vi "~ExampleCluster.vi"() -> ()   [LabVIEW 2017]
uses:
  Users/chris clark/Documents/Bolder/SEAKR/OBP/Product_Development/ULIP_SFP/LoopBackUtility/LoopbackToolClasses/ConfigMgr_N-ReceiverSubvis/Properties_N-Receiver.ctl
panel:
  in  "Replace? (F)":bool
  out "DefaultProperties out":T1={"Network"={"Local IP Address"="", "FPGA IP Address"="", "Local UDP Listener Port"=50000, "Destination UDP Port"=64880, "Rx Listener Timeout, ms"=0, "Receive Buffer Size"=8192, "Send Buffer Size"=512, "RemoteIPAddresses"=[]}, "TX Properties"={"Interpacket Gap, ms"=1, "Insert gap (N)"=1, "Packet.TxType"=0, "Packet.MaxLen"=8968, "Packet.MinLen"=7000}} {"TX Properties"."Packet.TxType" items=["Fixed", "Variable"]}
  in  "Write=True":bool
  in  "CfgFilePath":path=path "C:/dummy/testCluzzterz.ini"
  out "error out 2":errorcluster
  in  "DefaultProperties":T1={"Network"={"Local IP Address"="", "FPGA IP Address"="", "Local UDP Listener Port"=50000, "Destination UDP Port"=64880, "Rx Listener Timeout, ms"=0, "Receive Buffer Size"=8192, "Send Buffer Size"=512, "RemoteIPAddresses"=[]}, "TX Properties"={"Interpacket Gap, ms"=1, "Insert gap (N)"=1, "Packet.TxType"=0, "Packet.MaxLen"=8968, "Packet.MinLen"=7000}} {"TX Properties"."Packet.TxType" items=["Fixed", "Variable"]}
  # "Replace=True blows away\nold array values (deletes\nsections before writing)"
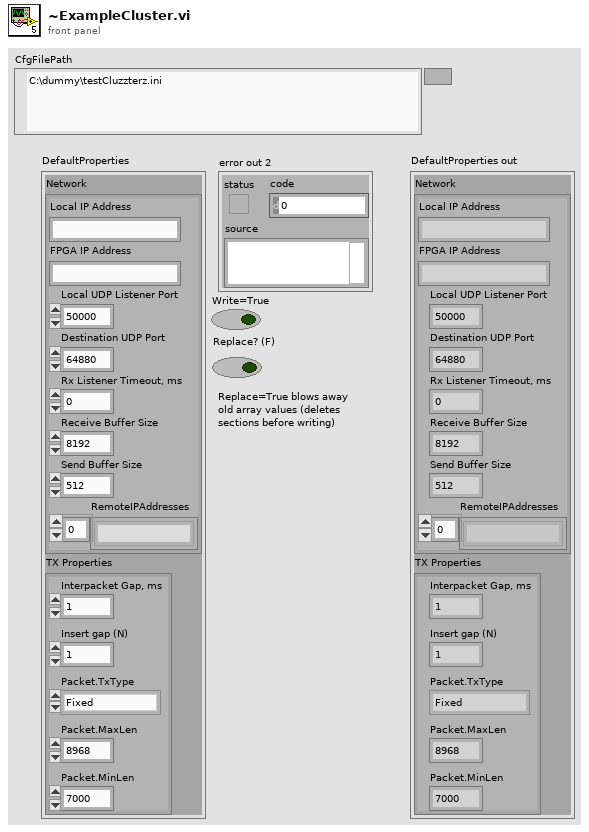
[diagram p1: front panel]
types:
  T1 = typedef "Properties_N-Receiver.ctl" = cluster{"Network":cluster{"Local IP Address":string, "FPGA IP Address":string, "Local UDP Listener Port":u16, "Destination UDP Port":u16, "Rx Listener Timeout, ms":i32, "Receive Buffer Size":u32, "Send Buffer Size":u32, "RemoteIPAddresses":string[]}, "TX Properties":cluster{"Interpacket Gap, ms":u32, "Insert gap (N)":i32, "Packet.TxType":i32, "Packet.MaxLen":i32, "Packet.MinLen":i32}}
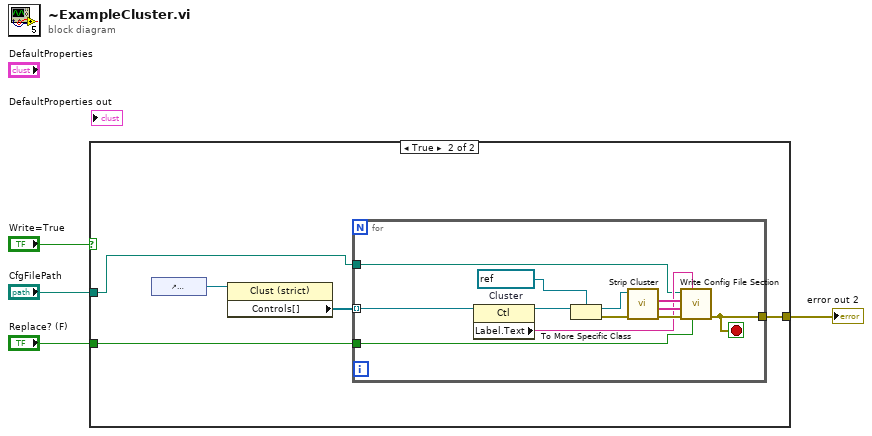
[diagram p0: block diagram]
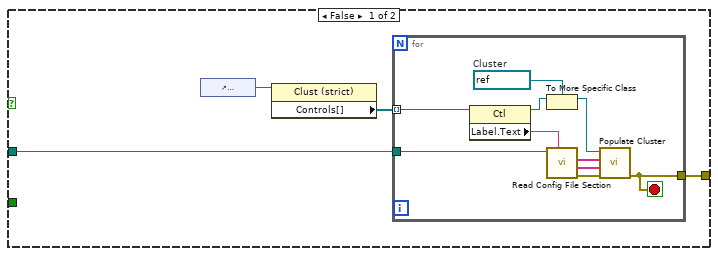
[diagram p2: hidden frame]
diagram:
  n1 = case shown="True" "Write=True" {
    tunnel: [w7 w23] -> w4
    tunnel: "CfgFilePath" -> [w8 w22]
    tunnel: "Replace? (F)" -> [_ w19]
    frame False {
      n2 = control-ref of="DefaultProperties out"() -> (w5:refnum<vi>)
      n3 = property class="Clust (strict)"(reference=w5) -> ("Controls[]"=w6:refnum<vi>[])  [unwired: 1 in, 2 out]
      n4 = for {
        tunnel: w6 -> [w18] mode=indexing
        tunnel: w8 -> [w16]
        tunnel: [w12] -> w7
        stop <- w12 stop-if-true
        w11 = refnum<vi> refnum  # Cluster
        n5 = property class="Ctl"(reference=w18) -> (reference out=w10:refnum<vi>, "Label.Text"=w17:string)  [unwired: 1 in, 1 out]
        n6 = To More Specific Class(target class=w11, reference=w10) -> (specific class reference=w9:refnum<vi>)  [unwired: 1 in, 1 out]
        n7 = call "Read Config File Section.vi"("Section"=w17, "appended path"=w16) -> ("error out"=w13:errorcluster, "Values"=w14:string[], "Keys"=w15:string[])  [unwired: 7 in]
        n8 = call "Populate Cluster.vi"("error in (no error)"=w13, "Values"=w14, "Keys"=w15, "Clust Refnum"=w9) -> ("error out"=w12:errorcluster)  [unwired: 6 in, 1 out]
      }
    }
    frame True {
      n9 = control-ref of="DefaultProperties"() -> (w21:refnum<vi>)
      n10 = property class="Clust (strict)"(reference=w21) -> ("Controls[]"=w20:refnum<vi>[])  [unwired: 1 in, 2 out]
      n11 = for {
        tunnel: w20 -> [w28] mode=indexing
        tunnel: [w29] -> w23
        tunnel: w22 -> [w25]
        tunnel: w19 -> [w24]
        stop <- w29 stop-if-true
        w35 = refnum<vi> refnum  # Cluster
        n12 = property class="Ctl"(reference=w28) -> (reference out=w27:refnum<vi>, "Label.Text"=w26:string)  [unwired: 1 in, 1 out]
        n13 = To More Specific Class(target class=w35, reference=w27) -> (specific class reference=w34:refnum<vi>, error out=w31:errorcluster)  [unwired: 1 in]
        n14 = call "Strip Cluster.vi"("error in (no error)"=w31, "Cluster Refnum"=w34) -> ("error out"=w30:errorcluster, "Values"=w32:string[], "Keys"=w33:string[])  [unwired: 6 in, 1 out]
        n15 = call "Write Config File Section.vi"("Replace? (F)"=w24, "Section"=w26, "error in"=w30, "Values"=w32, "Keys"=w33, "INI path"=w25) -> ("error out"=w29:errorcluster)  [unwired: 5 in]
      }
    }
  }
  "error out 2" <- w4
